vi "rs3 init api.vi"(8 "error in (no error)":errorcluster) -> (0 "error out":errorcluster, 2 "rscontext":u64=1752067024, 3 "api_version":i32=20710)   [LabVIEW 2023]
doc: "Initialized communication to the RealSense API. \n\nReturns:\nError Error text\nrscontext Context handle that needs to be used in INIT ALL\napi version The libRS API version number"
panel:
  # "RS3 Init API"
  # "(C) 2017 Intel Corp.,  AGJ"
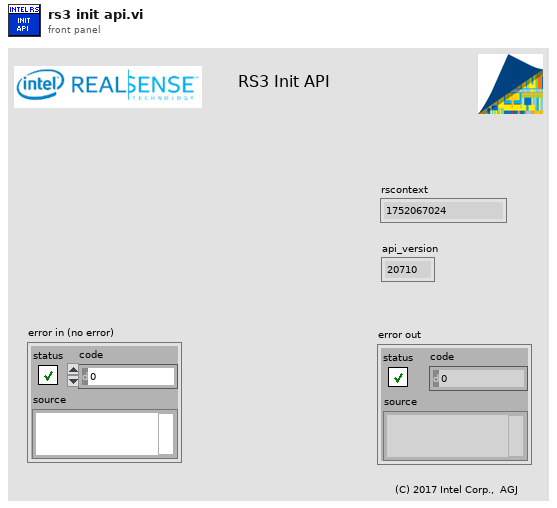
[diagram p1: front panel]
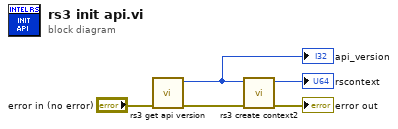
[diagram p0: block diagram]
diagram:
  n1 = call "rs3 get api version.vi"("error in (no error)"="error in (no error)") -> ("error out"=w4:errorcluster, "version"=w5:i32)  [unwired: 9 in]
  "api_version" <- w5
  n2 = call "rs3 create context2.vi"("error in (no error)"=w4, "version"=w5) -> ("error out"=→"error out":errorcluster, "context"=→"rscontext":u32)  [unwired: 8 in]
